vi "Data to DataBase.vi"(4 "Cost":u8, 6 "Name":string, 8 "error in (no error)":errorcluster, 9 "Datetime string":string, 10 "Database path":path, 11 "User Interface in":refnum<class "User Interface.lvclass">) -> (0 "error out":errorcluster, 3 "User Interface out":refnum<class "User Interface.lvclass">)   [LabVIEW 2020, in "User Interface.lvlib" / "User Interface.lvclass"]
uses:
  User Interface.lvclass
  User Interface.lvclass/User Interface.ctl
  Contabilidad/Contabilidad Messages/Update DataBase Msg/Update DataBase Msg.lvclass/Update DataBase Msg.ctl
  <vilib>/ActorFramework/Message Enqueuer/Message Enqueuer.lvclass/Message Enqueuer.ctl
  <vilib>/ActorFramework/Message Enqueuer/Enqueue.vi
  Contabilidad/Contabilidad Messages/Update DataBase Msg/Update DataBase Msg.lvclass
  C:/Program Files (x86)/National Instruments/LabVIEW 2020/vi.lib/ActorFramework/Message/Message.lvclass
  <vilib>/ActorFramework/Message Priority Queue/Priority Enqueue.vi
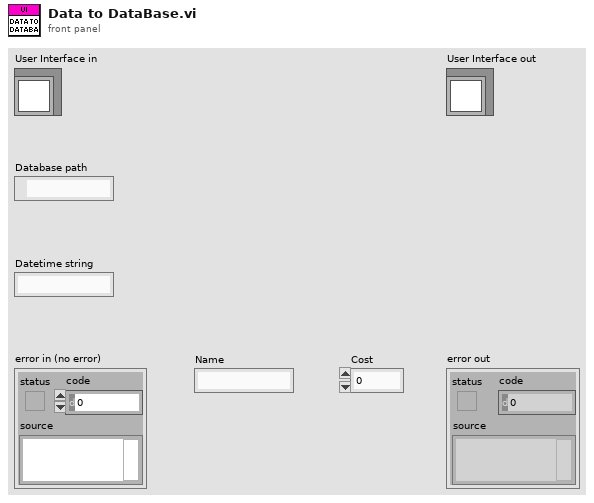
[diagram p1: front panel]
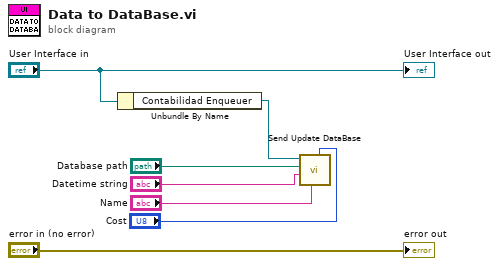
[diagram p0: block diagram]
diagram:
  n1 = Unbundle By Name("User Interface in") -> ("Contabilidad Enqueuer"=w5:refnum<class "Message Enqueuer.lvclass">)
  n2 = call "Send Update DataBase.vi"("Cost"="Cost", "Name"="Name", "Datetime string"="Datetime string", "Database path"="Database path", "Message Enqueuer"=w5) -> ()  [unwired: 5 in, 2 out]
  "error out" <- "error in (no error)"
  "User Interface out" <- "User Interface in"
